vi "Initialize Control.vi"(8 "error in (no error)":errorcluster, 11 "Cleaningcycle in":refnum<class "Cleaning cycle.lvclass">) -> (0 "error out":errorcluster, 3 "Cleaningcycle out":refnum<class "Cleaning cycle.lvclass">)   [LabVIEW 2016, in "Cleaning cycle.lvclass"]
doc: "The <b>Initialize VI</b> is a dynamic dispatch VI that must be overwritten in every QControl Class. It must <b>Call Parent Method</b> so that it recursively calls the initialize routine all of the way up the inheritance hierarchy. \n\nThe top most call is to the <b>Initialize Control VI</b> in Control.lvclass. This is the VI that starts the <b>Event Handler VI</b> if there was one overwritten in the QControl.\n<b> </b> <b> </b>\n©2016 Q Software Innovations, LLC (QSI)\nwritten by Quentin Alldredge\nproduced in LabVIEW 2015\n\nsupport@qsoftwareinnovations.com\nwww.qsoftwareinnovations.com\n\nAll rights reserved.\n\nRedistribution and use in source and binary forms, with or without modification, are permitted provided that the following conditions are met:\n\n * Redistributions of source code must retain the above copyright notice, this list of conditions and the following disclaimer.\n * Redistributions in binary form must reproduce the above copyright notice, this list of conditions and the following disclaimer in the documentation and/or other materials provided with the distribution.\n * Neither the name of Q Software Innovations, LLC. nor the names of its contributors may be used to endorse or promote products derived from this software without specific prior written permission.\n\nTHIS SOFTWARE IS PROVIDED BY THE COPYRIGHT HOLDERS AND CONTRIBUTORS \"AS IS\" AND ANY EXPRESS OR IMPLIED WARRANTIES, INCLUDING, BUT NOT LIMITED TO, THE IMPLIED WARRANTIES OF MERCHANTABILITY AND FITNESS FOR A PARTICULAR PURPOSE ARE DISCLAIMED. IN NO EVENT SHALL THE COPYRIGHT OWNER OR CONTRIBUTORS BE LIABLE FOR ANY DIRECT, INDIRECT, INCIDENTAL, SPECIAL, EXEMPLARY, OR CONSEQUENTIAL DAMAGES (INCLUDING, BUT NOT LIMITED TO, PROCUREMENT OF SUBSTITUTE GOODS OR SERVICES; LOSS OF USE, DATA, OR PROFITS; OR BUSINESS INTERRUPTION) HOWEVER CAUSED AND ON ANY THEORY OF LIABILITY, WHETHER IN CONTRACT, STRICT LIABILITY, OR TORT (INCLUDING NEGLIGENCE OR OTHERWISE) ARISING IN ANY WAY OUT OF THE USE OF THIS SOFTWARE, EVEN IF ADVISED OF THE POSSIBILITY OF SUCH DAMAGE."
uses:
  Cleaning cycle.lvclass
  <vilib>/QSI/QControls/QControl Classes/Cluster/Cluster.lvclass
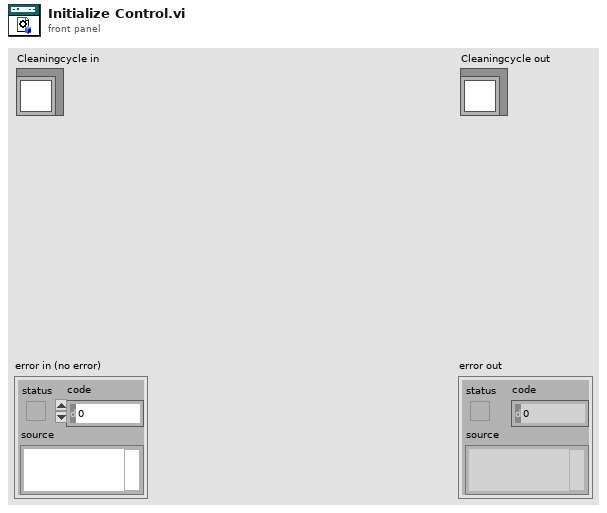
[diagram p1: front panel]
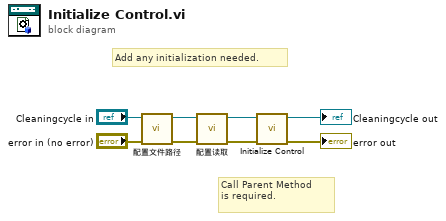
[diagram p0: block diagram]
diagram:
  # "Add any initialization needed."
  # "Call Parent Method\nis required."
  n1 = call "配置文件路径.vi"("error in (no error)"="error in (no error)", "Cleaningcycle 输入"="Cleaningcycle in") -> ("error out"=w2:errorcluster, "Cleaningcycle 输出"=w5:refnum<class "Cleaning cycle.lvclass">)  [unwired: 8 in]
  n2 = call "配置读取.vi"("error in (no error)"=w2, "Cleaningcycle 输入"=w5) -> ("error out"=w1:errorcluster, "Cleaningcycle 输出"=w4:refnum<class "Cleaning cycle.lvclass">)  [unwired: 8 in]
  n3 = call-parent "Initialize Control.vi"("error in (no error)"=w1, "Control in"=w4) -> ("error out"=→"error out":errorcluster, "Control out"=→"Cleaningcycle out":refnum<class "Cleaning cycle.lvclass">)  [unwired: 8 in]
